vi "Get ErrorCluster.vi"(8 "error in (no error)":errorcluster, 11 "ErrorMsg in":refnum<class "ErrorMsg.lvclass">) -> (0 "error out":errorcluster, 2 "ErrorCluster":errorcluster, 3 "ErrorMsg out":refnum<class "ErrorMsg.lvclass">)   [LabVIEW 2013, in "LapDog.Messaging.v3.lvlib" / "ErrorMsg.lvclass"]
doc: "Returns the error cluster contained in the error message.\n\nThis method executes regardless of the error in state."
uses:
  ErrorMsg.lvclass
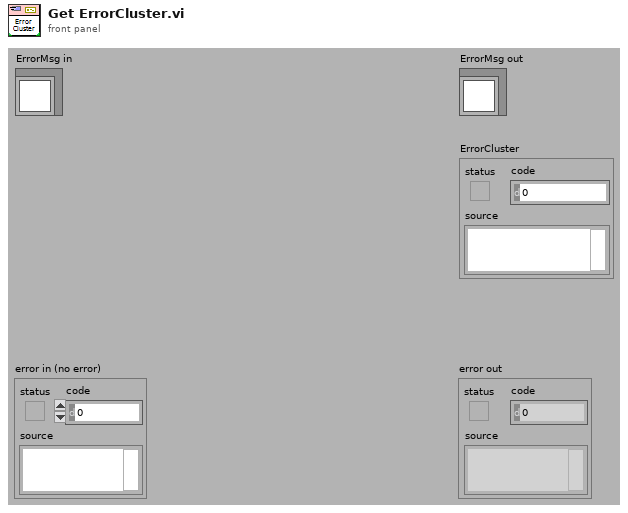
[diagram p1: front panel]
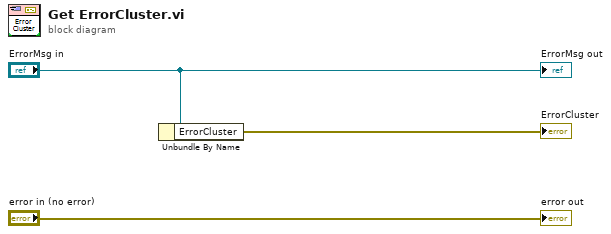
[diagram p0: block diagram]
diagram:
  n1 = Unbundle By Name("ErrorMsg in") -> ("ErrorCluster"=→"ErrorCluster":errorcluster)
  "error out" <- "error in (no error)"
  "ErrorMsg out" <- "ErrorMsg in"
